vi "PI_ScannerLine_In_Range.vi"(0 "Line Width":dbl=50.0 min=0.1 max=200.0 format="%1.1f um", 1 "Line Scan Axis":enum32{"x-Axis", "y-Axis", "z-Axis"}(ring) caption="Axis", 4 "Starting Point":T1) -> (14 "Line Width out":dbl=50.0 min=0.1 max=200.0 format="%1.1f um")   [LabVIEW 2010]
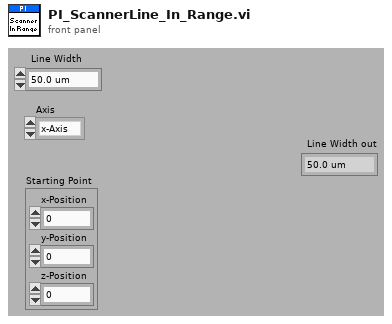
[diagram p1: front panel]
types:
  T1 = cluster{"x-Position":dbl, "y-Position":dbl, "z-Position":dbl}
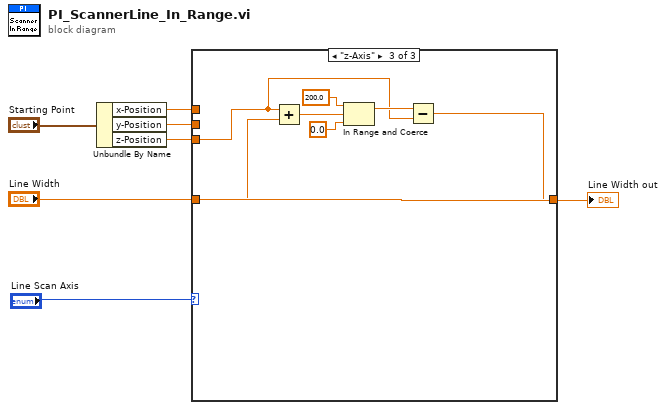
[diagram p0: block diagram]
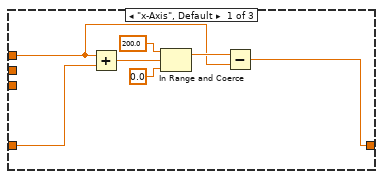
[diagram p2: hidden frame]
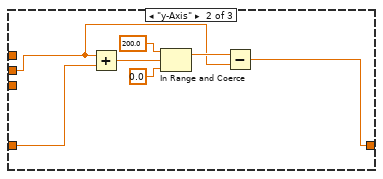
[diagram p3: hidden frame]
diagram:
  n1 = Unbundle By Name("Starting Point") -> ("x-Position"=w3:dbl, "y-Position"=w4:dbl, "z-Position"=w2:dbl)
  n2 = case shown="\"z-Axis\"" "Line Scan Axis" {
    tunnel: "Line Width" -> [w13 w20 w27]
    tunnel: w4 -> [_ w14 _]
    tunnel: w3 -> [w8 _ _]
    tunnel: w2 -> [_ _ w22]
    tunnel: [w7 w15 w23] -> _
    frame "x-Axis", Default {
      n3 = Add(x=w8, y=w13) -> (x+y=w12:dbl)
      n4 = In Range and Coerce(upper limit=200.0, x=w12, lower limit=0.0) -> (coerced(x)=w9:dbl)  [unwired: 1 out]
      n5 = Subtract(x=w9, y=w8) -> (x-y=w7:dbl)
    }
    frame "y-Axis" {
      n6 = Add(x=w14, y=w20) -> (x+y=w19:dbl)
      n7 = In Range and Coerce(upper limit=200.0, x=w19, lower limit=0.0) -> (coerced(x)=w16:dbl)  [unwired: 1 out]
      n8 = Subtract(x=w16, y=w14) -> (x-y=w15:dbl)
    }
    frame "z-Axis" {
      n9 = Add(x=w22, y=w27) -> (x+y=w26:dbl)
      n10 = In Range and Coerce(upper limit=200.0, x=w26, lower limit=0.0) -> (coerced(x)=w24:dbl)  [unwired: 1 out]
      n11 = Subtract(x=w24, y=w22) -> (x-y=w23:dbl)
    }
  }
  "Line Width out" <- "Line Width"
